vi "template.get.vi"(8 "error in":errorcluster, 11 "Client in":refnum<class "Client.lvclass">) -> (0 "error out":errorcluster, 3 "Client out":refnum<class "Client.lvclass">)   [LabVIEW 2020, in "Client.lvclass"]
doc: "Fetches a template by its rid and returns a handle to it."
uses:
  Client.lvclass
  Client.lvclass/Client.ctl
  client.lvlib
panel:
  out "out_template out":i32
  in  "rid":string
  in  "out_template":i32
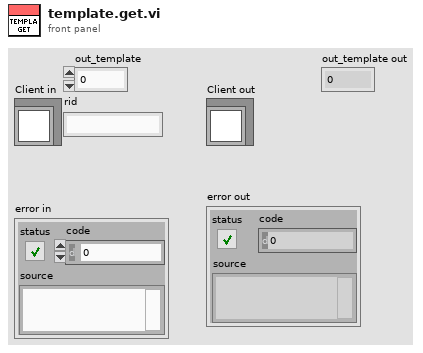
[diagram p1: front panel]
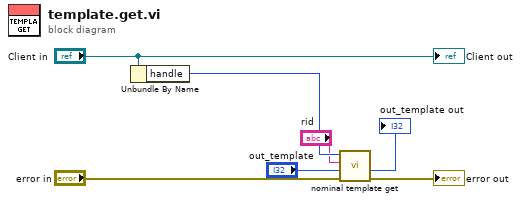
[diagram p0: block diagram]
diagram:
  n1 = Unbundle By Name("Client in") -> ("handle"=w5:i32)
  n2 = call "nominal template get.vi"("error in (no error)"="error in", "out_template"="out_template", "rid"="rid", "client"=w5) -> ("error out"=→"error out":errorcluster, "out_template out"=→"out_template out":i32)  [unwired: 5 in, 1 out]
  "Client out" <- "Client in"
